vi "Angle in degrees to u16.vi"(10 "angle to u16 scale factor":dbl, 11 "Angle (deg)":dbl) -> (2 "angle < 0?":bool, 3 "u16 angle":u16)   [LabVIEW 2015, in "Engine Simulation Toolkit Shared.lvlib"]
uses:
  Engine Simulation Toolkit Shared.lvlib
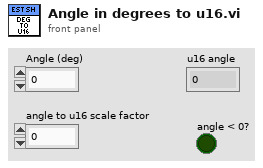
[diagram p1: front panel]
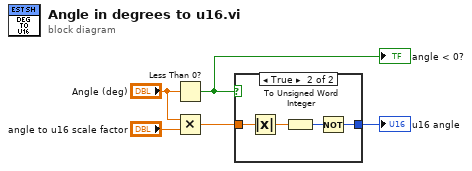
[diagram p0: block diagram]
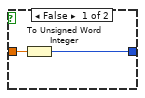
[diagram p2: hidden frame]
diagram:
  n1 = Less Than 0?(x="Angle (deg)") -> (x < 0?=w4:bool)
  "angle < 0?" <- w4
  n2 = Multiply(x="Angle (deg)", y="angle to u16 scale factor") -> (x*y=w3:dbl)
  n3 = case shown="True" w4 {
    tunnel: w3 -> [w7 w9]
    tunnel: [w6 w8] -> w2
    frame False {
      n4 = To Unsigned Word Integer(number=w7) -> (unsigned 16bit integer=w6:u16)
    }
    frame True {
      n5 = Absolute Value(x=w9) -> (abs(x)=w10:dbl)
      n6 = To Unsigned Word Integer(number=w10) -> (unsigned 16bit integer=w11:u16)
      n7 = Not(x=w11) -> (.not. x?=w8:u16)
    }
  }
  "u16 angle" <- w2
